vi "readGraphFromTDMS.vi"(0 "Refnum NumNb":refnum<vi>, 1 "Refnum en entrée":refnum<vi>, 5 "Error IN":errorcluster caption="constante d'erreur") -> (9 "YFP (°C)":cluster{"Y":dbl[], "Y":dbl[]}[](graph), 10 "Strip lue":string, 11 "YFP (s)":cluster{"Y":dbl[], "Y":dbl[]}[](graph), 12 "TEMPERATURE (°C)":cluster{"Y":dbl[], "Y":dbl[]}[](graph), 13 "LSSmOrange (°C)":cluster{"Y":dbl[], "Y":dbl[]}[](graph), 14 "CFP (s)":cluster{"Y":dbl[], "Y":dbl[]}[](graph), 15 "CFP (°C)":cluster{"Y":dbl[], "Y":dbl[]}[](graph), 16 "Error OUT":errorcluster caption="constante d'erreur", 17 "mAmétrine (s)":cluster{"Y":dbl[], "Y":dbl[]}[](graph), 18 "mAmétrine (°C)":cluster{"Y":dbl[], "Y":dbl[]}[](graph), 19 "LSSmOrange (s)":cluster{"Y":dbl[], "Y":dbl[]}[](graph))   [LabVIEW 2020]
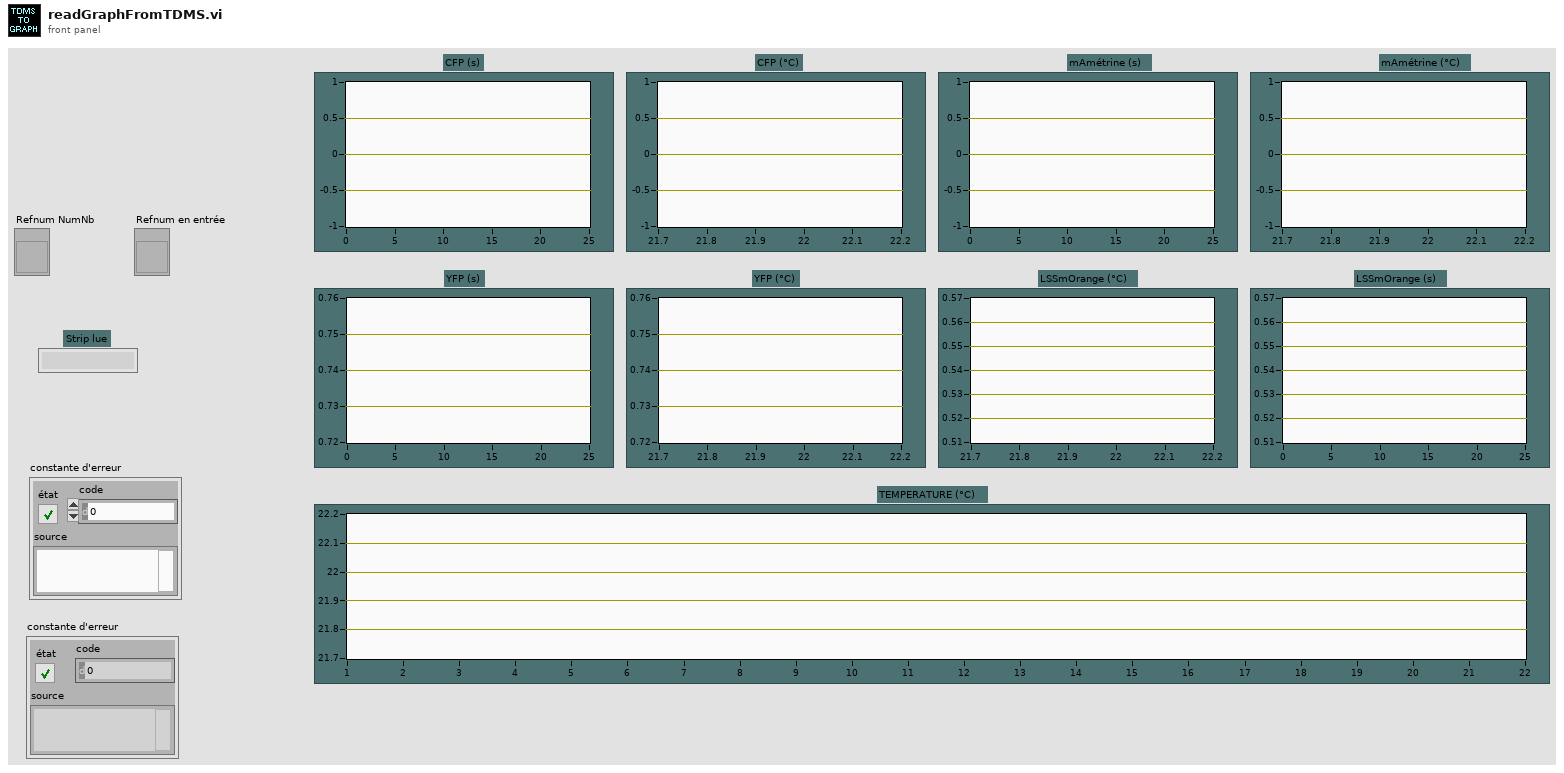
[diagram p1: front panel]
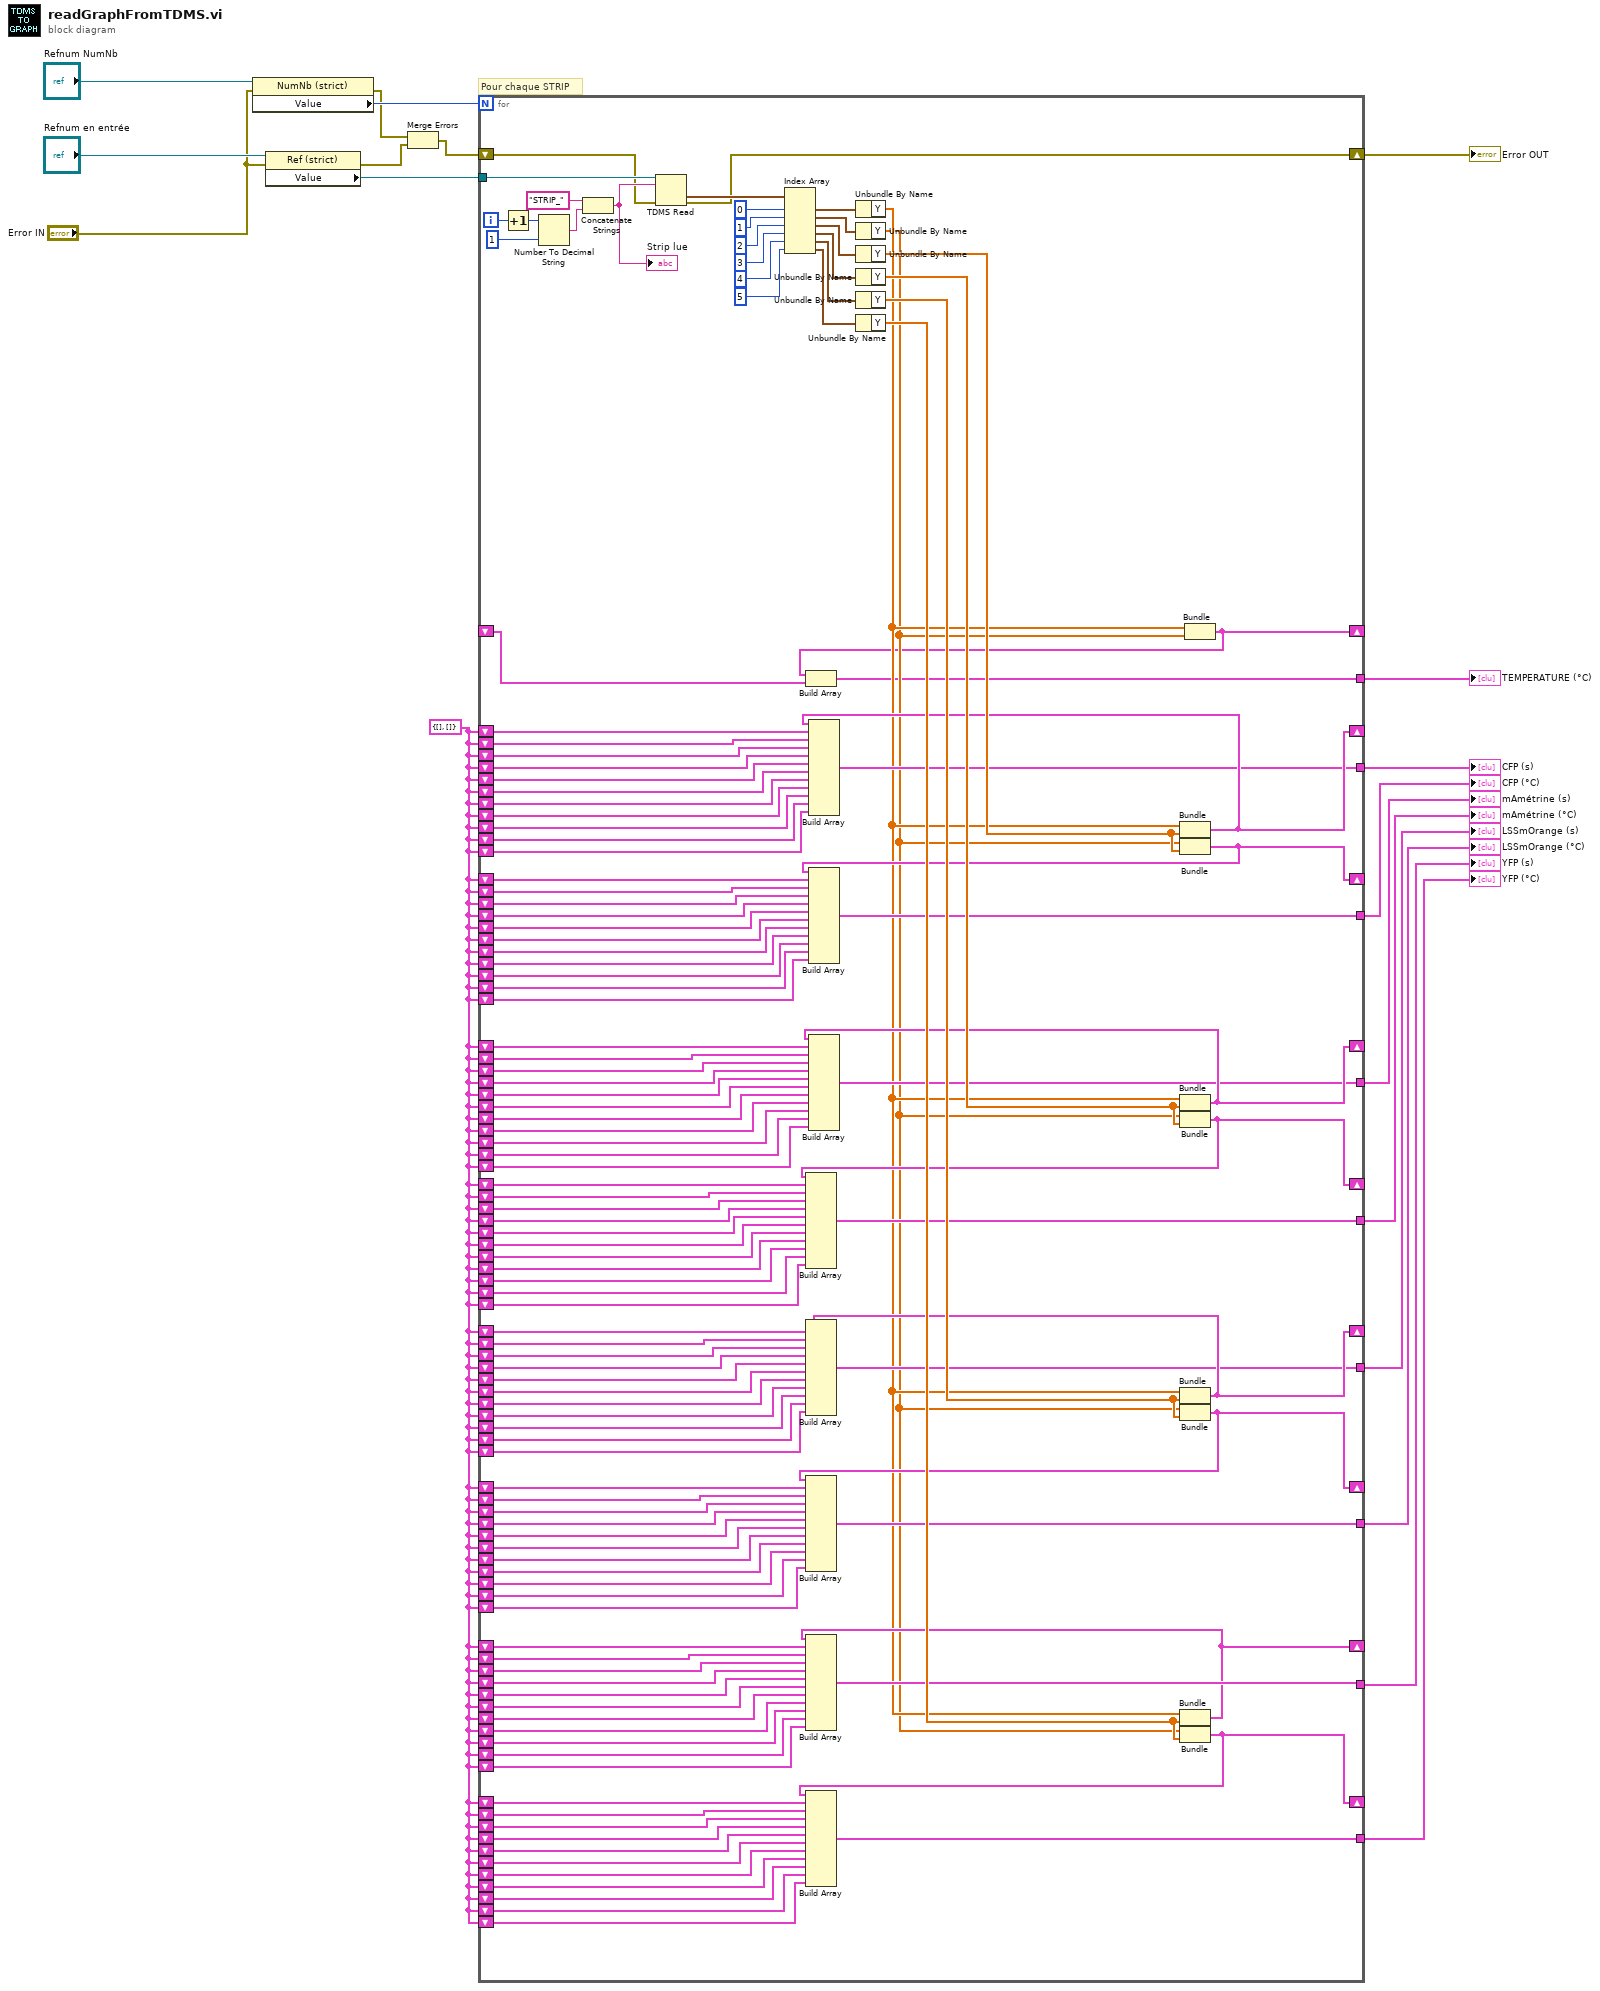
[diagram p0: block diagram]
diagram:
  w6 = cluster{dbl[], dbl[]} {[], []}
  # "Pour chaque STRIP"
  n1 = property on="Nœud de propriété" class="NumNb (strict)"(reference="Refnum NumNb", error in="Error IN") -> (error out=w4:errorcluster, "Value"=w16:i32)  [unwired: 1 out]
  n2 = property on="Nœud de propriété" class="Ref (strict)"(reference="Refnum en entrée", error in="Error IN") -> (error out=w3:errorcluster, "Value"=w15:refnum<k34>)  [unwired: 1 out]
  n3 = Merge Errors(w4, w3) -> (w1:errorcluster)
  n4 = for {
    N: w16 -> [_]
    tunnel: w15 -> [w139]
    shift-right: [w132] -> _
    shift-left: w6 -> [w129]
    shift-left: w6 -> [w128]
    shift-left: w6 -> [w127]
    shift-left: w6 -> [w126]
    shift-left: w6 -> [w125]
    shift-left: w6 -> [w124]
    shift-left: w6 -> [w123]
    shift-left: w6 -> [w122]
    shift-left: w6 -> [w121]
    shift-left: w6 -> [w120]
    shift-left: w6 -> [w119]
    shift-right: [w131] -> _
    shift-left: w6 -> [w118]
    shift-left: w6 -> [w117]
    shift-left: w6 -> [w116]
    shift-left: w6 -> [w115]
    shift-left: w6 -> [w114]
    shift-left: w6 -> [w113]
    shift-left: w6 -> [w112]
    shift-left: w6 -> [w111]
    shift-left: w6 -> [w110]
    shift-left: w6 -> [w109]
    shift-left: w6 -> [w108]
    tunnel: [w130] -> w14
    shift-right: [w96] -> _
    shift-left: w6 -> [w97]
    shift-left: w6 -> [w107]
    shift-left: w6 -> [w106]
    shift-left: w6 -> [w105]
    shift-left: w6 -> [w104]
    shift-left: w6 -> [w103]
    shift-left: w6 -> [w102]
    shift-left: w6 -> [w101]
    shift-left: w6 -> [w100]
    shift-left: w6 -> [w99]
    shift-left: w6 -> [w98]
    shift-right: [w95] -> _
    shift-left: w6 -> [w94]
    shift-left: w6 -> [w93]
    shift-left: w6 -> [w92]
    shift-left: w6 -> [w91]
    shift-left: w6 -> [w90]
    shift-left: w6 -> [w89]
    shift-left: w6 -> [w88]
    shift-left: w6 -> [w87]
    shift-left: w6 -> [w86]
    shift-left: w6 -> [w85]
    shift-left: w6 -> [w84]
    shift-right: [w61] -> _
    shift-left: w6 -> [w83]
    shift-right: [w60] -> _
    shift-left: w6 -> [w72]
    shift-left: w6 -> [w82]
    shift-left: w6 -> [w81]
    shift-left: w6 -> [w80]
    shift-left: w6 -> [w79]
    shift-left: w6 -> [w78]
    shift-left: w6 -> [w77]
    shift-left: w6 -> [w76]
    shift-left: w6 -> [w75]
    shift-left: w6 -> [w74]
    shift-left: w6 -> [w73]
    shift-left: w6 -> [w71]
    shift-left: w6 -> [w70]
    shift-left: w6 -> [w69]
    shift-left: w6 -> [w62]
    shift-left: w6 -> [w68]
    shift-left: w6 -> [w67]
    shift-left: w6 -> [w66]
    shift-left: w6 -> [w65]
    shift-left: w6 -> [w64]
    shift-left: w6 -> [w63]
    tunnel: [w59] -> w13
    tunnel: [w58] -> w12
    tunnel: [w57] -> w11
    tunnel: [w56] -> w10
    tunnel: [w55] -> w9
    shift-right: [w52] -> _
    shift-left: w6 -> [w50]
    shift-left: w6 -> [w49]
    shift-left: w6 -> [w48]
    shift-left: w6 -> [w47]
    shift-left: w6 -> [w46]
    shift-left: w6 -> [w45]
    shift-left: w6 -> [w44]
    shift-left: w6 -> [w43]
    shift-left: w6 -> [w42]
    shift-left: w6 -> [w41]
    shift-left: w6 -> [w40]
    shift-right: [w51] -> _
    shift-left: w6 -> [w39]
    tunnel: [w54] -> w7
    tunnel: [w53] -> w8
    shift-left: w6 -> [w38]
    shift-left: w6 -> [w37]
    shift-left: w6 -> [w36]
    shift-left: w6 -> [w35]
    shift-left: w6 -> [w34]
    shift-left: w6 -> [w33]
    shift-left: w6 -> [w32]
    shift-left: w6 -> [w31]
    shift-left: w6 -> [w30]
    shift-left: w6 -> [w29]
    tunnel: [w22] -> w5
    shift-right: [w23] -> _
    shift-left: _ -> [w24]
    shift-right: [w21] -> w2
    shift-left: w1 -> [w20]
    i -> [w153]
    n5 = Increment(x=w153) -> (x+1=w150:i32)
    n6 = Number To Decimal String(number=w150, width (-)=i16 1 ("largeur (-)")) -> (decimal integer string=w151:string)
    n7 = Concatenate Strings("STRIP_" ("nom du groupe en entrée"), w151) -> (w138:string)
    "Strip lue" <- w138
    n8 = TDMS Read(0:w139, 5:w138, 11:w20) -> (10:w137:waveform(dbl)[], 15:w21:errorcluster)  [unwired: 5 in, 4 out]
    n9 = Index Array(array=w137, index #1=0 ("indice"), index #2=1 ("indice"), index #3=2 ("indice"), index #4=3 ("indice"), index #5=4 ("indice"), index #6=5 ("indice")) -> (element #1=w145:waveform(dbl), element #2=w144:waveform(dbl), element #3=w143:waveform(dbl), element #4=w142:waveform(dbl), element #5=w141:waveform(dbl), element #6=w140:waveform(dbl))
    n10 = Unbundle By Name(w145) -> ("Y"=w28:dbl[])
    n11 = Unbundle By Name(w144) -> ("Y"=w27:dbl[])
    n12 = Unbundle By Name(w143) -> ("Y"=w136:dbl[])
    n13 = Unbundle By Name(w142) -> ("Y"=w135:dbl[])
    n14 = Unbundle By Name(w141) -> ("Y"=w134:dbl[])
    n15 = Unbundle By Name(w140) -> ("Y"=w133:dbl[])
    n16 = Bundle("Y"=w28, "Y"=w136) -> (w132:cluster{"Y":dbl[], "Y":dbl[]})  [unwired: 1 in]
    n17 = Build Array(w132, w129, w128, w127, w126, w125, w124, w123, w122, w121, w120, w119) -> (w130:cluster{"Y":dbl[], "Y":dbl[]}[])
    n18 = Bundle("Y"=w27, "Y"=w136) -> (w131:cluster{"Y":dbl[], "Y":dbl[]})  [unwired: 1 in]
    n19 = Build Array(w131, w118, w117, w116, w115, w114, w113, w112, w111, w110, w109, w108) -> (w59:cluster{"Y":dbl[], "Y":dbl[]}[])
    n20 = Bundle("Y"=w28, "Y"=w135) -> (w96:cluster{"Y":dbl[], "Y":dbl[]})  [unwired: 1 in]
    n21 = Build Array(w96, w97, w107, w106, w105, w104, w103, w102, w101, w100, w99, w98) -> (w58:cluster{"Y":dbl[], "Y":dbl[]}[])
    n22 = Bundle("Y"=w27, "Y"=w135) -> (w95:cluster{"Y":dbl[], "Y":dbl[]})  [unwired: 1 in]
    n23 = Build Array(w95, w94, w93, w92, w91, w90, w89, w88, w87, w86, w85, w84) -> (w57:cluster{"Y":dbl[], "Y":dbl[]}[])
    n24 = Bundle("Y"=w28, "Y"=w134) -> (w61:cluster{"Y":dbl[], "Y":dbl[]})  [unwired: 1 in]
    n25 = Build Array(w61, w83, w82, w81, w80, w79, w78, w77, w76, w75, w74, w73) -> (w56:cluster{"Y":dbl[], "Y":dbl[]}[])
    n26 = Bundle("Y"=w27, "Y"=w134) -> (w60:cluster{"Y":dbl[], "Y":dbl[]})  [unwired: 1 in]
    n27 = Build Array(w60, w72, w71, w70, w69, w62, w68, w67, w66, w65, w64, w63) -> (w55:cluster{"Y":dbl[], "Y":dbl[]}[])
    n28 = Bundle("Y"=w28, "Y"=w133) -> (w52:cluster{"Y":dbl[], "Y":dbl[]})  [unwired: 1 in]
    n29 = Build Array(w52, w50, w49, w48, w47, w46, w45, w44, w43, w42, w41, w40) -> (w54:cluster{"Y":dbl[], "Y":dbl[]}[])
    n30 = Bundle("Y"=w27, "Y"=w133) -> (w51:cluster{"Y":dbl[], "Y":dbl[]})  [unwired: 1 in]
    n31 = Build Array(w51, w39, w38, w37, w36, w35, w34, w33, w32, w31, w30, w29) -> (w53:cluster{"Y":dbl[], "Y":dbl[]}[])
    n32 = Bundle("Y"=w28, "Y"=w27) -> (w23:cluster{"Y":dbl[], "Y":dbl[]})  [unwired: 1 in]
    n33 = Build Array(w23, w24) -> (w22:cluster{"Y":dbl[], "Y":dbl[]}[])
  }
  "CFP (s)" <- w14
  "CFP (°C)" <- w13
  "mAmétrine (s)" <- w12
  "mAmétrine (°C)" <- w11
  "LSSmOrange (s)" <- w10
  "LSSmOrange (°C)" <- w9
  "YFP (s)" <- w7
  "YFP (°C)" <- w8
  "TEMPERATURE (°C)" <- w5
  "Error OUT" <- w2
